vi "onStopped.vi"(8 "error in (no error)":errorcluster, 11 "SMO":refnum<class "SMO.lvclass">) -> (0 "error out":errorcluster, 3 "SMO out":refnum<class "SMO.lvclass">)   [LabVIEW 2013, in "SMO.lvclass"]
uses:
  SMO.lvclass
  Typedefs/SMOState --Enum.ctl
  Typedefs/SMO Dependency Event--Cluster.ctl
  Typedefs/SMO Dependency Event--Enum.ctl
  Support/Attribute.Owner/Attribute.Owner.lvclass
  Support/Attribute.Dependencies/Attribute.Dependencies.lvclass
panel:
  # "For instructions on how to use the JKI State Machine Objects, examples and video tutorials, visit:\nhttp://jki.net/state-machine-objects/\n\nJKI State Machine Objects™\nhttp://jki.net/state-machine-objects/\nCopyright (C) 2005-2015, JKI <info@jki.net>\nALL RIGHTS RESERVED"
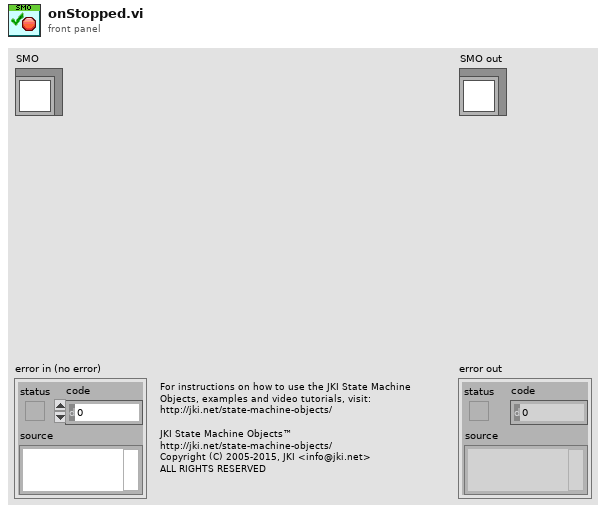
[diagram p1: front panel]
types:
  T1 = typedef "SMO.lvclass/SMOState --Enum.ctl" = enum16{"unknown", "Created", "Started", "Stopped"}
  T2 = typedef "SMOAttributes.lvlib/Attribute.Dependencies.lvclass/DependencyAttr--Cluster.ctl" = cluster{"Name":string, "GUID":string, "owned":bool, "shared":bool, "Level":string, "SMO":refnum<class "SMO.lvclass">}
  T3 = typedef "SMO.lvclass/SMO Dependency Event--Cluster.ctl" = cluster{"Name":string, "GUID":string, "Event":T4}
  T4 = typedef "SMO.lvclass/SMO Dependency Event--Enum.ctl" = enum16{"Added", "Removed", "Started", "Stopped"}
  T5 = typedef "SMO.lvclass/Protected Events.ctl" = cluster{"StopProcesses":refnum<user-event>, "AbortProcesses":refnum<user-event>, "Config Changed":refnum<user-event>, "Dependency":refnum<user-event>}
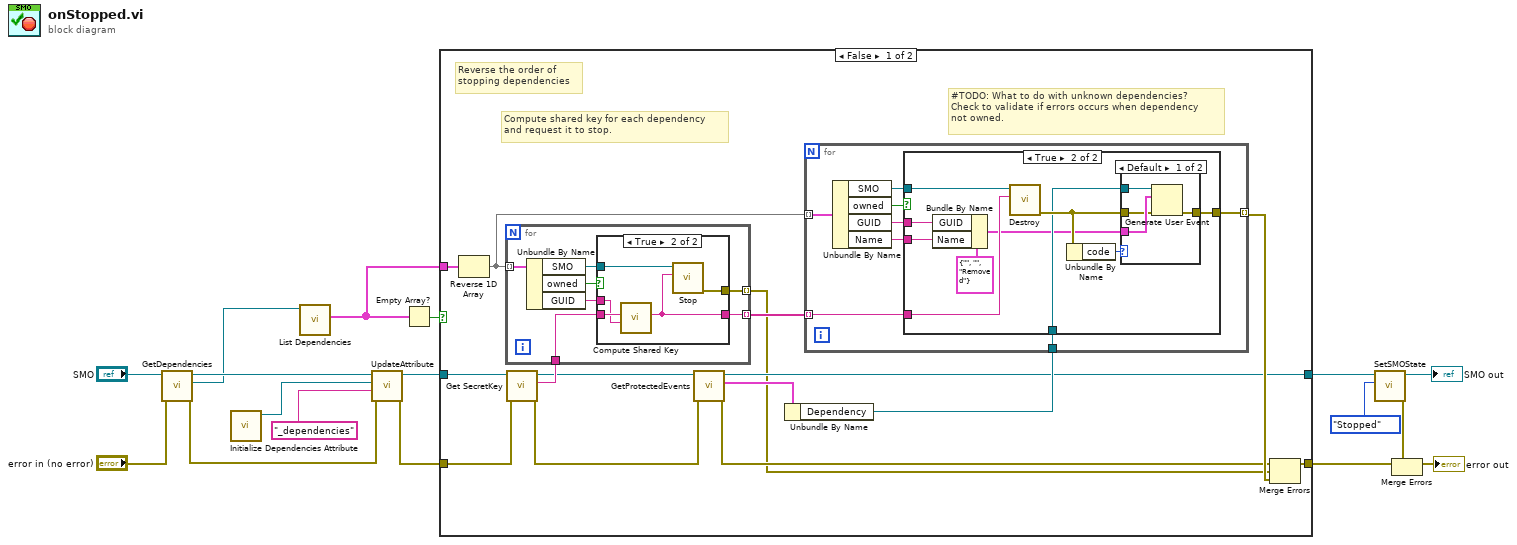
[diagram p0: block diagram]
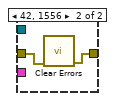
[diagram p3: hidden frame]
diagram:
  n1 = call "GetDependencies.vi"("error in (no error)"="error in (no error)", "SMO in"="SMO") -> ("error out"=w4:errorcluster, "Dependencies"=w7:refnum<class "Attribute.Dependencies.lvclass">, "SMO out"=w8:refnum<class "SMO.lvclass">)  [unwired: 7 in]
  n2 = call "Initialize Dependencies Attribute.vi"() -> ("Attribute.Dependencies"=w10:refnum<class "Attribute.Dependencies.lvclass">)  [unwired: 11 in]
  n3 = call "List Dependencies.vi"("Attribute.Dependencies in"=w7) -> ("Dependencies"=w5:T2[])  [unwired: 8 in, 2 out]
  n4 = call "UpdateAttribute.vi"("error in (no error)"=w4, "Attribute Name"="_dependencies" ("name"), "Attribute"=w10, "SMO in"=w8) -> ("error out"=w3:errorcluster, "SMO in"=w2:refnum<class "SMO.lvclass">)  [unwired: 5 in, 1 out]
  n5 = Empty Array?(array=w5) -> (empty?=w11:bool)
  n6 = case shown="False" w11 {
    tunnel: [w32 w69] -> w12
    tunnel: w5 -> [w31 _]
    tunnel: w2 -> [w30 w70]
    tunnel: w3 -> [w29 w69]
    tunnel: [w20 w70] -> w14
    frame False {
      # "#TODO: What to do with unknown dependencies?\nCheck to validate if errors occurs when dependency\nnot owned."
      # "Reverse the order of\nstopping dependencies"
      # "Compute shared key for each dependency\nand request it to stop."
      n7 = Reverse 1D Array(array=w31) -> (reversed array=w19:T2[])
      n8 = call "Get SecretKey.vi"("error in (no error)"=w29, "SMO"=w30) -> ("error out"=w24:errorcluster, "SecretKey"=w28:string, "SMO out"=w25:refnum<class "SMO.lvclass">)  [unwired: 7 in]
      n9 = for {
        tunnel: w19 -> [w62] mode=indexing
        tunnel: w28 -> [w63]
        tunnel: [w61] -> w27 mode=indexing
        tunnel: [w57] -> w18 mode=indexing
        n10 = Unbundle By Name(w62) -> ("SMO"=w58:refnum<class "SMO.lvclass">, "owned"=w59:bool, "GUID"=w60:string)
        n11 = case shown="True" w59 {
          tunnel: w63 -> [_ w68]
          tunnel: [_ w65] -> w61
          tunnel: w60 -> [_ w67]
          tunnel: w58 -> [_ w66]
          tunnel: [_ w64] -> w57
          frame False {
          }
          frame True {
            n12 = call "Compute Shared Key.vi"("GUID"=w67, "SecretKey"=w68) -> ("Shared Key"=w65:string)  [unwired: 9 in]
            n13 = call "Stop.vi"("Shared Key"=w65, "SMO"=w66) -> ("error out"=w64:errorcluster)  [unwired: 8 in, 1 out]
          }
        }
      }
      n14 = call "GetProtectedEvents.vi"("error in (no error)"=w24, "SMO"=w25) -> ("error out"=w23:errorcluster, "SMO Protected Events"=w22:T5, "SMO out"=w20:refnum<class "SMO.lvclass">)  [unwired: 7 in]
      n15 = Unbundle By Name(w22) -> ("Dependency"=w21:refnum<user-event>)
      n16 = for {
        tunnel: w27 -> [w40] mode=indexing
        tunnel: [w39] -> w26 mode=indexing
        tunnel: w21 -> [w38]
        tunnel: w19 -> [w37] mode=indexing
        n17 = Unbundle By Name(w37) -> ("SMO"=w36:refnum<class "SMO.lvclass">, "owned"=w33:bool, "GUID"=w35:string, "Name"=w34:string)
        n18 = case shown="True" w33 {
          tunnel: w40 -> [_ w50]
          tunnel: [_ w47] -> w39
          tunnel: w38 -> [_ w46]
          tunnel: w36 -> [_ w45]
          tunnel: w35 -> [_ w44]
          tunnel: w34 -> [_ w43]
          frame False {
          }
          frame True {
            n19 = Bundle By Name(cluster=T3 {"Name"="", "GUID"="", "Event"=enum."Removed"} ("Dependency Event"), "GUID"=w44, "Name"=w43) -> (w42:T3)
            n20 = call "Destroy.vi"("Shared Key"=w50, "SMO"=w45) -> ("error out"=w48:errorcluster)  [unwired: 9 in]
            n21 = Unbundle By Name(w48) -> ("code"=w49:i32)
            n22 = case shown="Default" w49 {
              tunnel: w48 -> [w52 w56]
              tunnel: [w51 w55] -> w47
              tunnel: w42 -> [w53 _]
              tunnel: w46 -> [w54 _]
              frame Default {
                n23 = Generate User Event(user event=w54, event data cluster=w53, error in=w52) -> (error out=w51:errorcluster)  [unwired: 1 in, 1 out]
              }
              frame 42, 1556 {
                n24 = call <vilib>:"Clear Errors.vi"("error in (no error)"=w56) -> ("error out"=w55:errorcluster)  [unwired: 6 in]
              }
            }
          }
        }
      }
      n25 = Merge Errors(w23, w18, w26) -> (w32:errorcluster)
    }
    frame True {
    }
  }
  n26 = call "SetSMOState.vi"("SMO State"=SMOState_--Enum."Stopped" ("event data"), "SMO in"=w14) -> ("error out"=w16:errorcluster, "SMO out"=→"SMO out":refnum<class "SMO.lvclass">)  [unwired: 8 in]
  n27 = Merge Errors(w12, w16) -> (→"error out":errorcluster)
